vi "Get Goal Node Reference.vi"(8 "error in (no error)":errorcluster, 11 "Anytime D* in":refnum<class "NI_Robotics_AnytimeDStar.lvclass">) -> (0 "error out":errorcluster, 2 "goal node reference":refnum<data-value>, 3 "Anytime D* out":refnum<class "NI_Robotics_AnytimeDStar.lvclass">)   [LabVIEW 2017, in "NI_Robotics_AnytimeDStar.lvclass"]
uses:
  <vilib>/robotics/Navigation/Anytime D Star/NI_Robotics_AnytimeDStar.lvclass
  <vilib>/robotics/Navigation/shared/MapNode/AbstractDstarNode/NI_Robotics_AbstractDstarNode.lvclass
  <vilib>/robotics/Navigation/Anytime D Star/NI_Robotics_AnytimeDStar.lvclass/NI_Robotics_AnytimeDStar.ctl
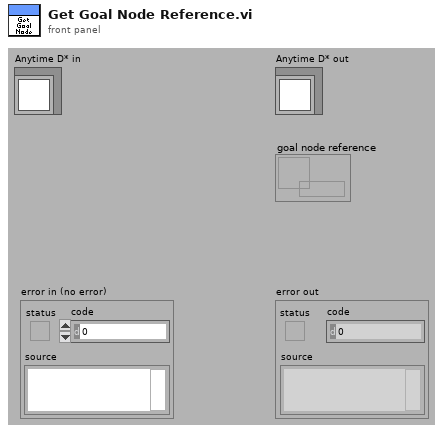
[diagram p1: front panel]
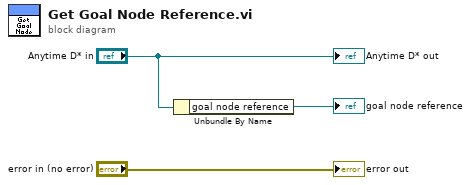
[diagram p0: block diagram]
diagram:
  n1 = Unbundle By Name("Anytime D* in") -> ("goal node reference"=→"goal node reference":refnum<data-value>)
  "Anytime D* out" <- "Anytime D* in"
  "error out" <- "error in (no error)"
